vi "kinectRead [ColorFrame].vi"(8 "Error In":errorcluster, 9 "Timeout (ms)":i32=5000, 11 "KinectSensor References in":T1) -> (0 "Error Out":errorcluster, 2 "frameData":u32[](array[numeric]), 3 "KinectSensor References out":T1)   [LabVIEW 2011, in "LVH-KinectOne.lvlib"]
doc: "Reads a color frame and returns the frame data. The frame data is returned as a 1-D array of unsigned 8 bit integers. Every 4 bytes corresponds to a pixel in RGBA format. The default resolution in pixels is 1920x1080."
uses:
  LVH-KinectOne.lvlib
  Type Defs/KinectSensor References.ctl
  Microsoft.Kinect
  C:/github/makerhub/KinectOne/LabVIEW/vi.lib/MakerHub/KinectOne/Private/Libs/BodyFrameDataInterface.dll
  Libs/BodyFrameDataInterface.dll
  Frame Data FGV [Color].vi
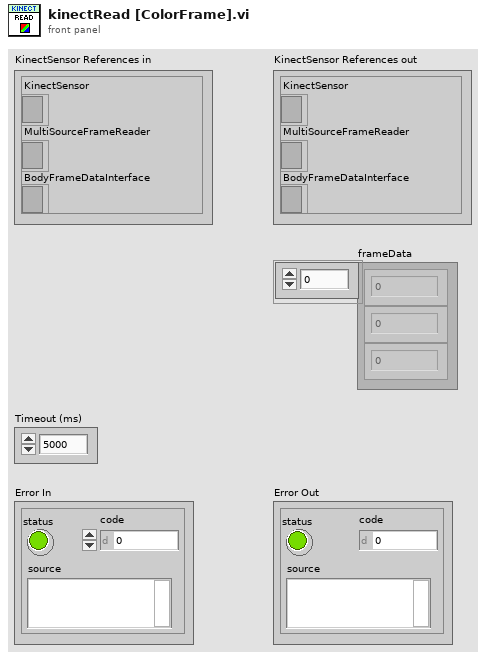
[diagram p1: front panel]
types:
  T1 = typedef "LVH-KinectOne.lvlib/KinectSensor References.ctl" = cluster{"KinectSensor":refnum<k24>, "MultiSourceFrameReader":refnum<k24>, "BodyFrameDataInterface":refnum<k24>}
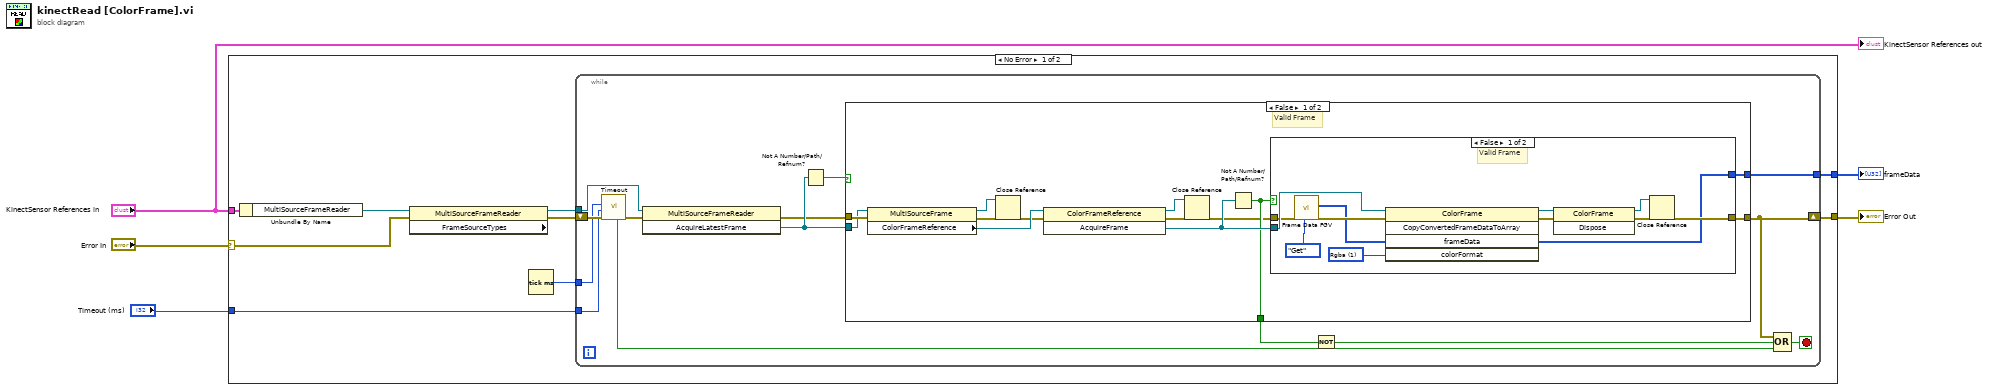
[diagram p0: block diagram]
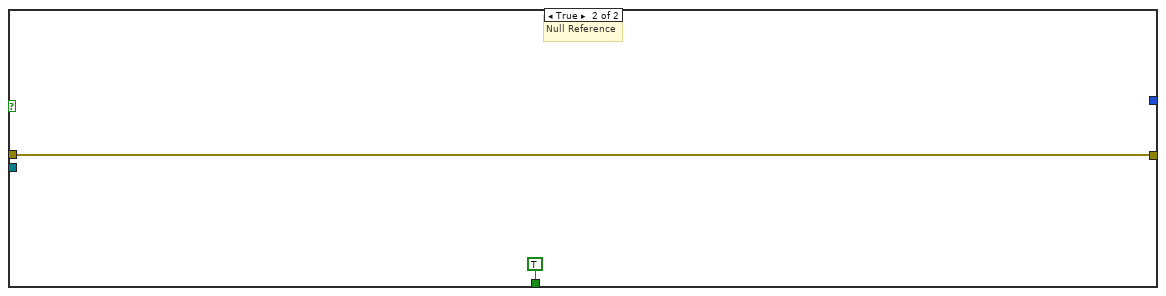
[diagram p3: hidden frame]
diagram:
  n1 = case shown="No Error" "Error In" {
    selector: "Error In" -> [w6 w57]
    tunnel: "KinectSensor References in" -> [w11 _]
    tunnel: [w10 w57] -> w4
    tunnel: [w9 _] -> w3
    tunnel: "Timeout (ms)" -> [w7 _]
    frame No Error {
      n2 = Unbundle By Name(w11) -> ("MultiSourceFrameReader"=w12:refnum<k24>)
      n3 = property class="MultiSourceFrameReader" props=["FrameSourceTypes"](reference=w12, error in=w6) -> (reference out=w14:refnum<k24>, error out=w13:errorcluster)  [unwired: 1 out]
      n4 = Tick Count (ms)() -> (millisecond timer value=w8:u32)
      n5 = while {
        tunnel: w14 -> [w23]
        shift-right: [w20] -> w10
        shift-left: w13 -> [w25]
        tunnel: [w26] -> w9
        tunnel: w8 -> [w22]
        tunnel: w7 -> [w21]
        stop <- w19 stop-if-true
        n6 = call "Timeout.vi"("error in (no error)"=w25, "Timeout (ms)"=w21, "Start Time"=w22) -> ("error out"=w24:errorcluster, "Timeout?"=w16:bool)  [unwired: 7 in]
        n7 = invoke class="MultiSourceFrameReader" method="AcquireLatestFrame"(reference=w23, error in=w24) -> (error out=w15:errorcluster, "AcquireLatestFrame"=w28:refnum<k24>)  [unwired: 1 in, 1 out]
        n8 = Not A Number/Path/Refnum?(number/path/refnum=w28) -> (NaN/Path/Refnum?=w27:bool)
        n9 = case shown="False" w27 {
          tunnel: w15 -> [w40 w55]
          tunnel: w28 -> [w37 _]
          tunnel: [w39 w55] -> w20
          tunnel: [w38 TRUE] -> w18
          tunnel: [w35 _] -> w26
          frame False {
            # "Valid Frame"
            n10 = property class="MultiSourceFrame"(reference=w37, error in=w40) -> (reference out=w33:refnum<k24>, error out=w34:errorcluster, "ColorFrameReference"=w36:refnum<k24>)
            n11 = Close Reference(reference=w33, error in (no error)=w34) -> (error out=w32:errorcluster)
            n12 = invoke class="ColorFrameReference" method="AcquireFrame"(reference=w36, error in=w32) -> (reference out=w30:refnum<k24>, error out=w31:errorcluster, "AcquireFrame"=w41:refnum<k24>)  [unwired: 1 in]
            n13 = Close Reference(reference=w30, error in (no error)=w31) -> (error out=w29:errorcluster)
            n14 = Not A Number/Path/Refnum?(number/path/refnum=w41) -> (NaN/Path/Refnum?=w38:bool)
            n15 = case shown="False" w38 {
              tunnel: w29 -> [w45 w54]
              tunnel: w41 -> [w48 _]
              tunnel: [w47 w54] -> w39
              tunnel: [w46 _] -> w35
              frame False {
                w49 = 1 items=["None", "Rgba", "Yuv", "Bgra", "Bayer", "Yuy2"] ("colorFormat")
                # "Valid Frame"
                n16 = call-poly "Frame Data FGV.vi"("Command"=enum16{"Get", "Initialize"}."Get", "error in (no error)"=w45) -> ("error out"=w44:errorcluster, "Byte Array"=w43:u8[])  [unwired: 8 in]
                n17 = invoke class="ColorFrame" method="CopyConvertedFrameDataToArray"(reference=w48, error in=w44, "frameData"=w43, "colorFormat"=w49) -> (reference out=w50:refnum<k24>, error out=w51:errorcluster, "frameData"=w46:u8[])  [unwired: 1 in, 2 out]
                n18 = invoke class="ColorFrame" method="Dispose"(reference=w50, error in=w51) -> (reference out=w53:refnum<k24>, error out=w52:errorcluster)  [unwired: 1 in, 1 out]
                n19 = Close Reference(reference=w53, error in (no error)=w52) -> (error out=w47:errorcluster)
              }
              frame True {
                # "Null Reference"
              }
            }
          }
          frame True {
            # "Null Reference"
          }
        }
        n20 = Not(x=w18) -> (.not. x?=w17:bool)
        n21 = Compound Arithmetic op=OR(w20, w17, w16) -> (w19:bool)
      }
    }
    frame Error {
    }
  }
  "Error Out" <- w4
  "frameData" <- w3
  "KinectSensor References out" <- "KinectSensor References in"
